vi "网络地址字符串 转 IP端口.vi"(6 "分隔符(:)":string=":", 11 "IP端口字符串":string) -> (3 "IP端口":cluster{"IP":string, "Port":u16})   [LabVIEW 2017]
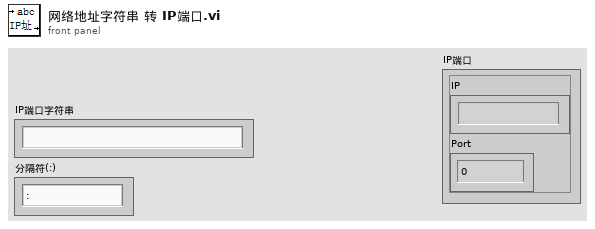
[diagram p1: front panel]
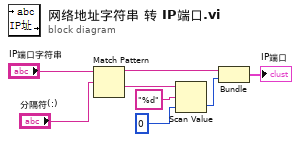
[diagram p0: block diagram]
diagram:
  n1 = Match Pattern(string="IP端口字符串", regular expression="分隔符(:)") -> (before substring=w3:string, after substring=w5:string)  [unwired: 1 in, 2 out]
  n2 = Scan Value(string=w5, format string="%d" ("格式字符串"), default (0 dbl)=u16 0 ("默认(0 dbl)")) -> (value=w4:u16)  [unwired: 1 out]
  n3 = Bundle("IP端口字符串"=w3, "默认(0 dbl)"=w4) -> (→"IP端口":cluster{"IP端口字符串":string, "默认(0 dbl)":u16})  [unwired: 1 in]
